vi "Delete document.vi"(8 "error in (no error)":errorcluster caption="entrée d'erreur (pas d'erreur)", 11 "Firebase (Default) en entrée":refnum<class "Firebase Driver.lvclass">) -> (0 "error out":errorcluster caption="sortie d'erreur", 3 "Firebase (Default) en sortie":refnum<class "Firebase Driver.lvclass">)   [LabVIEW 2020, in "Library Instrument & Equipement.lvlib" / "Library FireBase.lvlib" / "Firebase Driver.lvclass"]
uses:
  Firebase Driver.lvclass
  Commun VI/TypeDef/Liste Error.ctl
  Firebase Driver.lvclass/Firebase Driver.ctl
  JSON API/JSON Value/Set from JSON string.vi
  JSON API/JSON Value/JSON Value.lvclass
  JSON API/Get Polymorphic/JSON GetSet.lvlib
  <vilib>/httpClient/LabVIEWHTTPClient.lvlib
  JSON API/Variant JSON/Variant JSON.lvlib
  Commun VI/Library Commun.lvlib
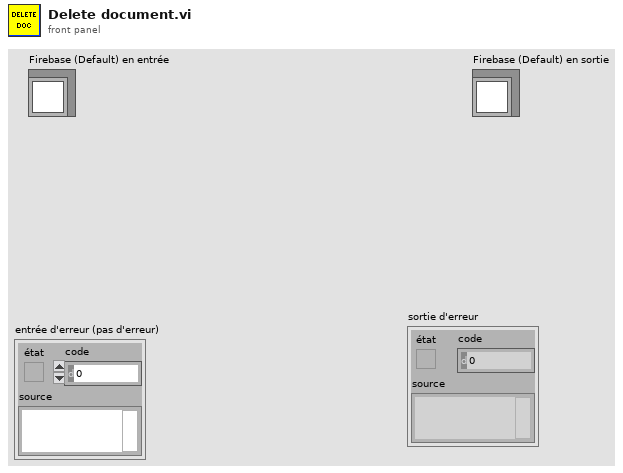
[diagram p1: front panel]
types:
  T1 = typedef "Library Commun.lvlib/Liste Error.ctl" = enum16{"Firebase Driver - Get Document", "Firebase Driver - Get Document With Where", "Firebase Driver - Delete Document", "Firebase Driver - Set Document", "Firebase Driver - Update Document", "Firebase Altyor - Search Document Bench", "Firebase Altyor - Class Not in Firebase", "Spectrum_Analyser - Timeout", "Relay Board - Qty Relay", "DIO - Pb Funtion", "Power_Supply - Peripherical not find", "Mutimeter - Peripherical not find", "Instrument - Function Not Used", "Instrument - Instrument name not specified", "Instrument - Allready Initialised", "Instrument - TimeOut", "Instrument - the instrument must be Initialise before", "Instrument - Frame Not received", "Instrument - Frame Nok", "Test - Initialise the File_for_Save", "Test - Timeout", "Test - Cmd Error", "FGV - Variable ", "BDD FireBase - Define Class", "SN - Class Not Define"}
  T2 = typedef "LabVIEWHTTPClient.lvlib/ClientHandle.ctl" = refnum<k1>
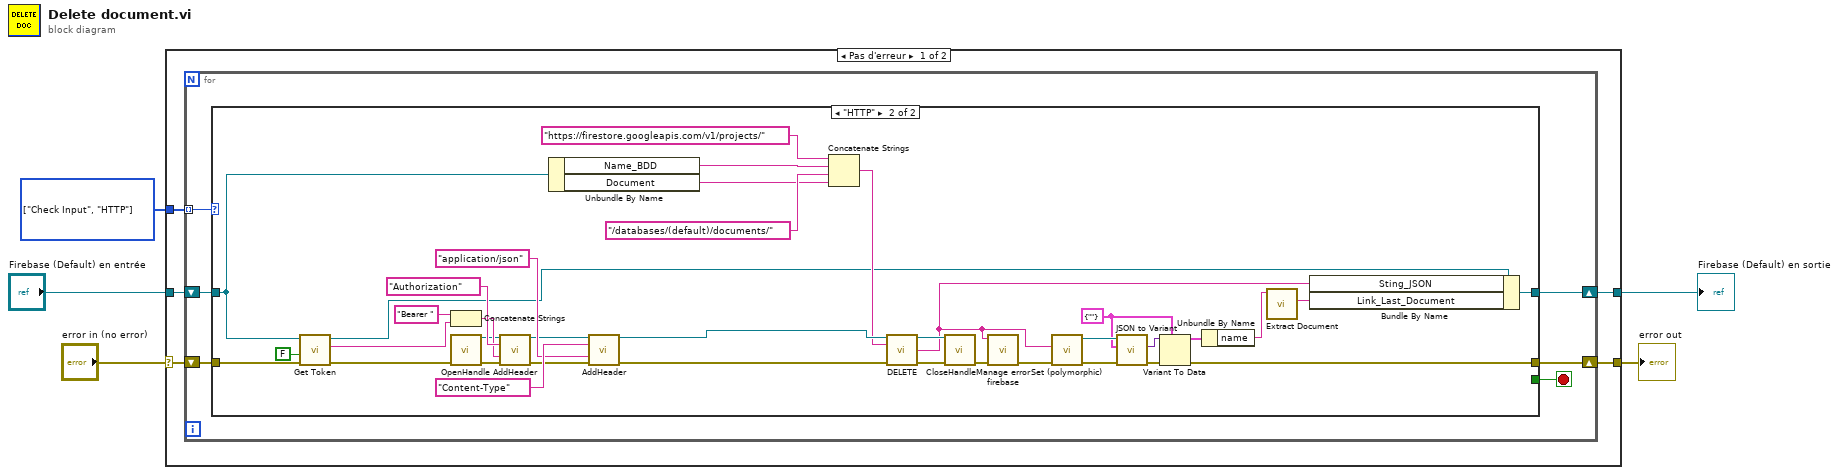
[diagram p0: block diagram]
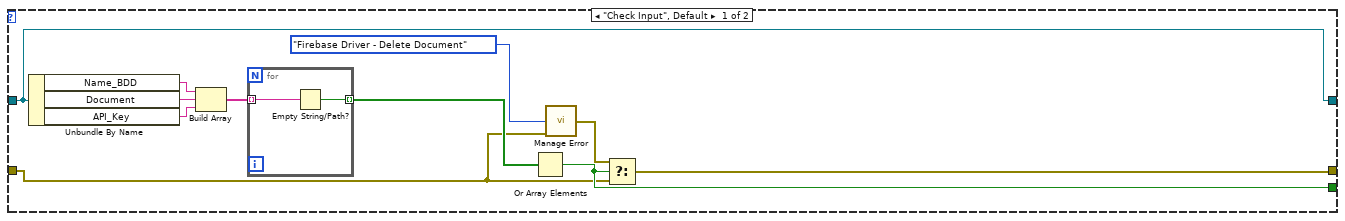
[diagram p2: hidden frame]
diagram:
  w1 = enum16{"Check Input", "HTTP"}[] [enum."Check Input", enum."HTTP"] items=["Check Input", "HTTP"]
  n1 = case shown="Pas d'erreur" "error in (no error)" {
    selector: "error in (no error)" -> [w10 w68]
    tunnel: [w9 w68] -> w4
    tunnel: "Firebase (Default) en entrée" -> [w8 w67]
    tunnel: [w7 w67] -> w2
    tunnel: w1 -> [w6 _]
    frame No Error {
      n2 = for {
        shift-right: [w13] -> w9
        shift-left: w10 -> [w16]
        shift-right: [w14] -> w7
        shift-left: w8 -> [w15]
        tunnel: w6 -> [w12] mode=indexing
        stop <- w11 stop-if-true
        n3 = case shown="\"HTTP\"" w12 {
          tunnel: w16 -> [w17 w51]
          tunnel: w15 -> [w23 w36]
          tunnel: [w23 w48] -> w14
          tunnel: [w24 w39] -> w13
          tunnel: [w25 _] -> w11
          frame "Check Input", Default {
            n4 = Unbundle By Name(w23) -> ("Name_BDD"=w22:string, "Document"=w21:string, "API_Key"=w20:string)
            n5 = Build Array(w22, w21, w20) -> (w27:string[])
            n6 = for {
              tunnel: w27 -> [w28] mode=indexing
              tunnel: [w29] -> w26 mode=indexing
              n7 = Empty String/Path?(string/path=w28) -> (empty?=w29:bool)
            }
            n8 = Or Array Elements(Boolean array=w26) -> (logical OR=w25:bool)
            n9 = call "Manage Error.vi"("Code Erreur"=Liste_Error."Firebase Driver - Delete Document", "error in (no error)"=w17) -> ("error out"=w18:errorcluster)  [unwired: 13 in]
            n10 = Select(t=w18, s=w25, f=w17) -> (s? t:f=w24:errorcluster)
          }
          frame "HTTP" {
            w43 = cluster{"name":string} {"name"=""}
            n11 = call-dynamic "Get Token.vi"("error in (no error)"=w51, "Reset"=FALSE, "Build Library FireBase.lvlib:Firebase (Default) IN"=w36) -> ("error out"=w50:errorcluster, "idToken"=w37:string, "Build Library FireBase.lvlib:Firebase (Default) Out"=w35:refnum<class "Firebase Driver.lvclass">)  [unwired: 6 in]
            n12 = Concatenate Strings("Bearer " ("chaîne"), w37) -> (w57:string)
            n13 = call <vilib>:"OpenHandle.vi"("error in (no error)"=w50) -> ("client handle out"=w55:T2, "error out"=w56:errorcluster)  [unwired: 13 in]
            n14 = call <vilib>:"AddHeader.vi"("client handle"=w55, "header"="Authorization", "value"=w57, "error in (no error)"=w56) -> ("client handle out"=w60:T2, "error out"=w61:errorcluster)  [unwired: 10 in]
            n15 = Unbundle By Name(w36) -> ("Name_BDD"=w52:string, "Document"=w34:string)
            n16 = call <vilib>:"AddHeader.vi"("client handle"=w60, "header"="Content-Type", "value"="application/json", "error in (no error)"=w61) -> ("client handle out"=w53:T2, "error out"=w32:errorcluster)  [unwired: 10 in]
            n17 = Concatenate Strings("https://firestore.googleapis.com/v1/projects/" ("string"), w52, "/databases/(default)/documents/" ("string"), w34) -> (w38:string)
            n18 = call <vilib>:"DELETE.vi"("client handle"=w53, "url"=w38, "error in (no error)"=w32) -> ("client handle out"=w64:T2, "body"=w31:string, "error out"=w65:errorcluster)  [unwired: 9 in, 1 out]
            n19 = call <vilib>:"CloseHandle.vi"("client handle"=w64, "error in (no error)"=w65) -> ("error out"=w54:errorcluster)  [unwired: 13 in]
            n20 = call "Manage error firebase.vi"("error in (no error)"=w54, "Body"=w31) -> ("error out"=w40:errorcluster)  [unwired: 9 in]
            n21 = call-poly "Set (polymorphic).vi"("error in (no error)"=w40, "JSON stream"=w31) -> ("error out"=w44:errorcluster, "JSON Value out"=w47:refnum<class "JSON Value.lvclass">)  [unwired: 7 in, 1 out]
            n22 = call "JSON to Variant.vi"("error in (no error)"=w44, "Variant (Data Type)"=w43, "JSON Value"=w47) -> ("error out"=w45:errorcluster, "Variant out"=w46:variant)  [unwired: 7 in]
            n23 = Variant To Data(error in=w45, type=w43, Variant=w46) -> (data=w42:cluster{"name":string}, error out=w39:errorcluster)
            n24 = Unbundle By Name(w42) -> ("name"=w41:string)
            n25 = call "Extract Document.vi"("Name"=w41) -> ("Source"=w33:string)  [unwired: 9 in, 1 out]
            n26 = Bundle By Name(cluster=w35, "Sting_JSON"=w31, "Link_Last_Document"=w33) -> (w48:refnum<class "Firebase Driver.lvclass">)
          }
        }
      }
    }
    frame Error {
    }
  }
  "error out" <- w4
  "Firebase (Default) en sortie" <- w2
